vi "ADC Checker.vi"(0 "Pump Data":T1={"Voltages"=[0.015201568603515625, 0.00335693359375, 0.003021240234375, 0.12260055541992188, 0.06085968017578125, 0.052234649658203125], "PumpCurrent"=[0.015201568603515625, 0.00335693359375, 0.003021240234375, 0.12260055541992188, 0.06085968017578125, 0.052234649658203125], "Speed"=[0.0, 0.0, 0.0, 0.0, 0.0, 0.0], "ControllerCurrent"=[0.015201568603515625, 0.00335693359375, 0.003021240234375, 0.12260055541992188, 0.06085968017578125, 0.052234649658203125], "Pressure"=[0.015201568603515625, 0.00335693359375, 0.003021240234375, 0.12260055541992188, 0.06085968017578125, 0.052234649658203125], "Flow"=[0.0, 0.0, 0.0, 0.125, 0.0625, 0.0625], "Elapsed Time (Display)"=[7.1, 7.1, 7.1, 458133.45, 458138.85000000003, 458126.75], "Avg Pressure"=0.0, "Avg Speed"=0.0, "Elapsed Time"=[4074.9003000000002, 4074.9003000000002, 4074.9003000000002, 4074.9003000000002, 4074.9003000000002, 4074.9003000000002]} {"Elapsed Time" format="%<%H:%M:%S>t"; "Elapsed Time (Display)" format="%<%H:%M:%S>t"; "Speed" format="%#_4f"; "ControllerCurrent" format="%#.1g"; "Pressure" format="%#.0f"; "Flow" format="%#.0f"; "PumpCurrent" format="%#.1g"; "Voltages" format="%#.0f"}, 5 "Run Profile":bool, 7 "Pumps Present":bool[](array[boolean]), 9 "Not Stopped":bool[](array[boolean])) -> (4 "Reset ADCs":bool)   [LabVIEW 2018]
uses:
  Controls/Pump Data.ctl
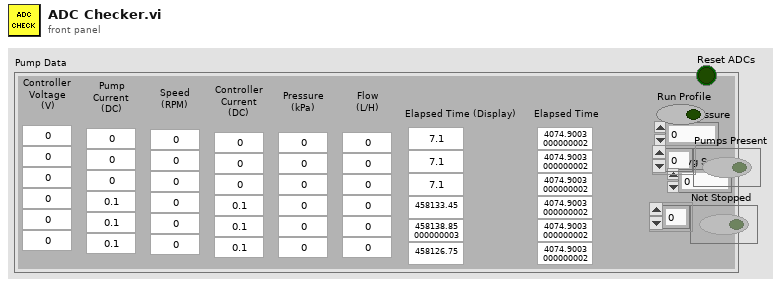
[diagram p1: front panel]
types:
  T1 = typedef "Pump Data.ctl" = cluster{"Voltages":dbl[], "PumpCurrent":dbl[], "Speed":dbl[], "ControllerCurrent":dbl[], "Pressure":dbl[], "Flow":dbl[], "Elapsed Time (Display)":dbl[], "Avg Pressure":dbl, "Avg Speed":dbl, "Elapsed Time":dbl[]}
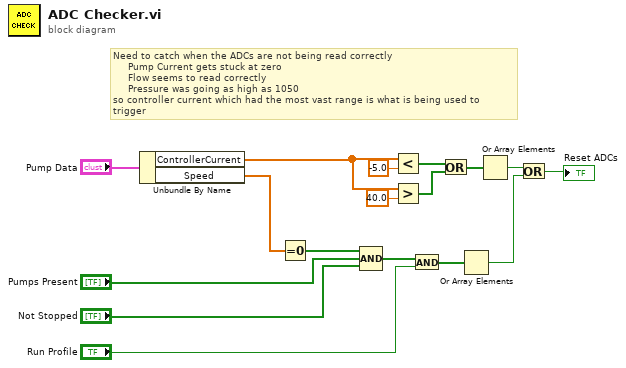
[diagram p0: block diagram]
diagram:
  # "Need to catch when the ADCs are not being read correctly\n     Pump Current gets stuck at zero\n     Flow seems to read correctly\n     Pressure was going as high as 1050\nso controller current which had the most vast range is what is being used to trigger"
  n1 = Unbundle By Name("Pump Data") -> ("ControllerCurrent"=w16:dbl[], "Speed"=w10:dbl[])
  n2 = Equal To 0?(x=w10) -> (x = 0?=w9:bool[])
  n3 = Compound Arithmetic op=AND(w9, "Pumps Present", "Not Stopped") -> (w6:bool[])
  n4 = Less?(x=w16, y=-5.0) -> (x < y?=w15:bool[])
  n5 = Greater?(x=w16, y=40.0) -> (0:w14:bool[])
  n6 = And(x=w6, y="Run Profile") -> (x .and. y?=w4:bool[])
  n7 = Or(x=w15, y=w14) -> (x .or. y?=w11:bool[])
  n8 = Or Array Elements(Boolean array=w4) -> (logical OR=w2:bool)
  n9 = Or Array Elements(Boolean array=w11) -> (logical OR=w3:bool)
  n10 = Or(x=w3, y=w2) -> (x .or. y?=→"Reset ADCs":bool)
